vi "Create CPU Monitor Frame from Standard Out.vi"(11 "Standard Output":string) -> (3 "Frame":variant)   [LabVIEW 2023]
uses:
  Type Definitions/Payload Class.ctl
  Type Definitions/Enumerated Constants/Software Monitor.ctl
  Type Definitions/CPU Usage.ctl
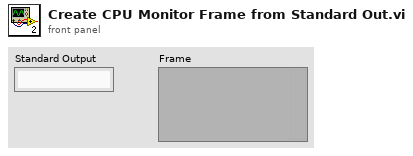
[diagram p1: front panel]
types:
  T1 = typedef "CPU Usage.ctl" = cluster{"User CPU Usage":sgl, "System CPU Usage":sgl, "NIC CPU ":sgl, "IO CPU Usage":sgl, "IRQ CPU Usage":sgl, "SIRQ CPU Usage":sgl, "Idle CPU Time":sgl}
  T2 = typedef "Software Monitor.ctl" = enum16{"Internet Connection Monitor", "CPU Monitor", "Archive Monitor", "Memory Monitor", "Queue Monitor", "RTOS Update", "RTOS Monitor"}
  T3 = typedef "Payload Class.ctl" = enum16{"System State", "Parameters", "Metadata", "Software Monitor", "Data", "Commands"}
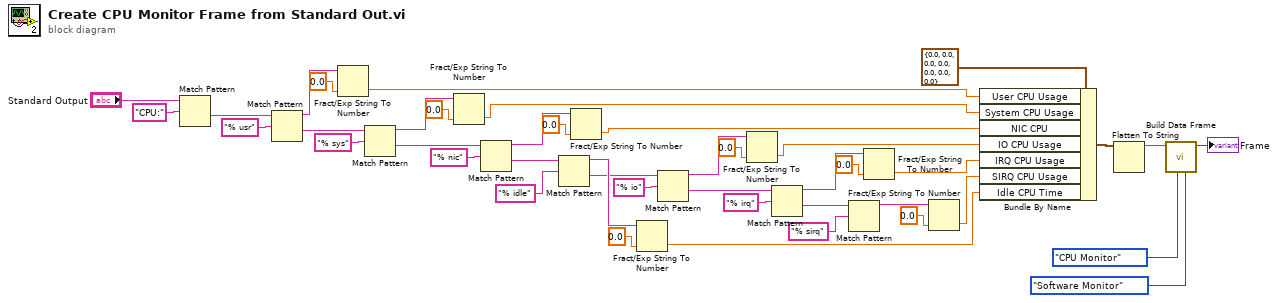
[diagram p0: block diagram]
diagram:
  n1 = Match Pattern(string="Standard Output", regular expression="CPU:") -> (after substring=w8:string)  [unwired: 1 in, 3 out]
  n2 = Match Pattern(string=w8, regular expression="% usr") -> (before substring=w22:string, after substring=w10:string)  [unwired: 1 in, 2 out]
  n3 = Fract/Exp String To Number(string=w22, default (0 dbl)=sgl 0.0 ("default (0 DBL)")) -> (number=w36:sgl)  [unwired: 2 in, 1 out]
  n4 = Match Pattern(string=w10, regular expression="% sys") -> (before substring=w29:string, after substring=w12:string)  [unwired: 1 in, 2 out]
  n5 = Fract/Exp String To Number(string=w29, default (0 dbl)=sgl 0.0 ("default (0 DBL)")) -> (number=w37:sgl)  [unwired: 2 in, 1 out]
  n6 = Match Pattern(string=w12, regular expression="% nic") -> (before substring=w30:string, after substring=w14:string)  [unwired: 1 in, 2 out]
  n7 = Match Pattern(string=w14, regular expression="% idle") -> (before substring=w31:string, after substring=w16:string)  [unwired: 1 in, 2 out]
  n8 = Fract/Exp String To Number(string=w30, default (0 dbl)=sgl 0.0 ("default (0 DBL)")) -> (number=w38:sgl)  [unwired: 2 in, 1 out]
  n9 = Fract/Exp String To Number(string=w31, default (0 dbl)=sgl 0.0 ("default (0 DBL)")) -> (number=w42:sgl)  [unwired: 2 in, 1 out]
  n10 = Match Pattern(string=w16, regular expression="% io") -> (before substring=w32:string, after substring=w19:string)  [unwired: 1 in, 2 out]
  n11 = Fract/Exp String To Number(string=w32, default (0 dbl)=sgl 0.0 ("default (0 DBL)")) -> (number=w39:sgl)  [unwired: 2 in, 1 out]
  n12 = Match Pattern(string=w19, regular expression="% irq") -> (before substring=w33:string, after substring=w20:string)  [unwired: 1 in, 2 out]
  n13 = Match Pattern(string=w20, regular expression="% sirq") -> (before substring=w34:string)  [unwired: 1 in, 3 out]
  n14 = Fract/Exp String To Number(string=w33, default (0 dbl)=sgl 0.0 ("default (0 DBL)")) -> (number=w40:sgl)  [unwired: 2 in, 1 out]
  n15 = Fract/Exp String To Number(string=w34, default (0 dbl)=sgl 0.0 ("default (0 DBL)")) -> (number=w41:sgl)  [unwired: 2 in, 1 out]
  n16 = Bundle By Name(cluster=T1 {"User CPU Usage"=0.0, "System CPU Usage"=0.0, "NIC CPU "=0.0, "IO CPU Usage"=0.0, "IRQ CPU Usage"=0.0, "SIRQ CPU Usage"=0.0, "Idle CPU Time"=0.0}, "User CPU Usage"=w36, "System CPU Usage"=w37, "NIC CPU"=w38, "IO CPU Usage"=w39, "IRQ CPU Usage"=w40, "SIRQ CPU Usage"=w41, "Idle CPU Time"=w42) -> (w4:T1)
  n17 = Flatten To String(anything=w4) -> (data string=w5:string)  [unwired: 3 in, 2 out]
  n18 = call "Build Data Frame.vi"("Payload Class (Data)"=Payload_Class."Software Monitor", "Payload ID (0)"=Software_Monitor."CPU Monitor", "Payload (Empty String)"=w5) -> ("Frame"=→"Frame":variant)  [unwired: 7 in, 1 out]
